vi "Main.vi"() -> ()   [LabVIEW 2020]
uses:
  Prime_Sieve/Prime_Sieve.lvclass
panel:
  out "Result":string
  out "Passes":i32
  in  "Size":i64=1000000
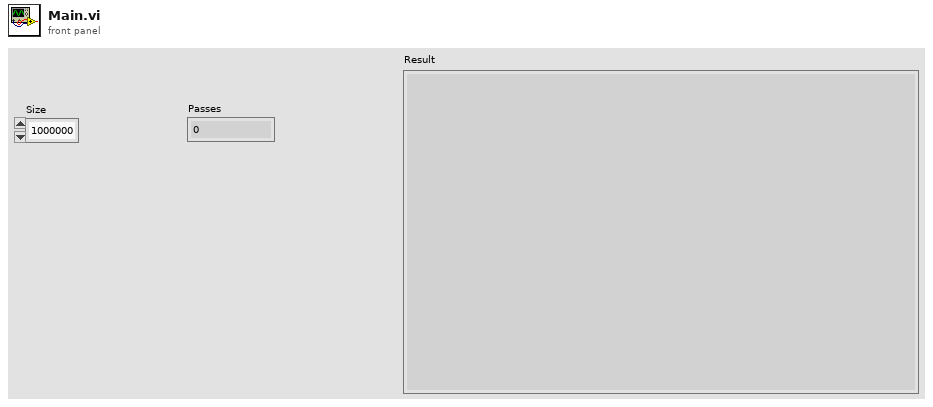
[diagram p1: front panel]
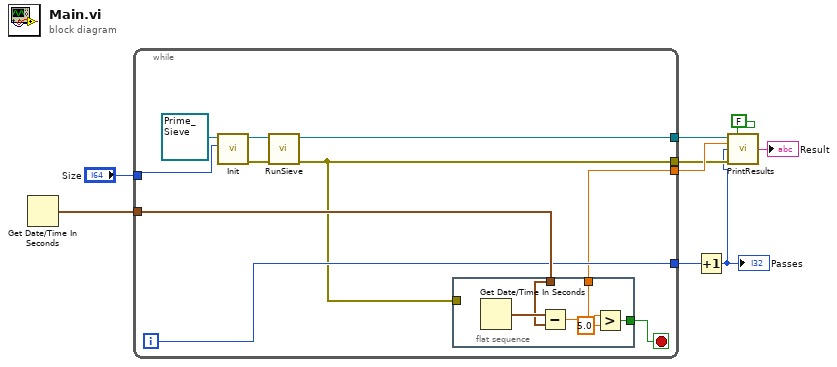
[diagram p0: block diagram]
diagram:
  n1 = Get Date/Time In Seconds() -> (seconds since 1Jan1904=w9:timestamp)
  n2 = while {
    tunnel: w9 -> [w19]
    tunnel: [w14] -> w8
    tunnel: "Size" -> [w13]
    tunnel: [w12] -> w6
    tunnel: [w11] -> w5
    tunnel: [w10] -> w4
    i -> [w14]
    stop <- w18 stop-if-true
    n3 = call "Init.vi"("Size"=w13, "Prime_Sieve in"=refnum<class "Prime_Sieve.lvclass"> refnum) -> ("error out"=w15:errorcluster, "Prime_Sieve out"=w16:refnum<class "Prime_Sieve.lvclass">)  [unwired: 8 in]
    n4 = call "RunSieve.vi"("error in (no error)"=w15, "Prime_Sieve in"=w16) -> ("error out"=w10:errorcluster, "Prime_Sieve out"=w12:refnum<class "Prime_Sieve.lvclass">)  [unwired: 8 in]
    n5 = flat-sequence {
      tunnel: w19 -> [w23]
      tunnel: [w21] -> w18
      tunnel: [w20] -> w11
      tunnel: w10 -> [_]
      frame #0 {
        n6 = Get Date/Time In Seconds() -> (seconds since 1Jan1904=w24:timestamp)
        n7 = Subtract(x=w24, y=w23) -> (x-y=w20:dbl)
        n8 = Greater?(x=w20, y=5.0) -> (0:w21:bool)
      }
    }
  }
  n9 = Increment(x=w8) -> (x+1=w2:i32)
  "Passes" <- w2
  n10 = call "PrintResults.vi"("Prime_Sieve in"=w6, "Show Results"=FALSE, "Duration"=w5, "Passes"=w2, "error in (no error)"=w4) -> ("Result"=→"Result":string)  [unwired: 8 in, 2 out]
